vi "获取仪器仪表状态.vi"(11 "站号":u16(ring)=3 items=["总磷"=1, "总氮"=2, "氨氮"=3, "CODMn"=21, "CODcr"=22]) -> (3 "工作状态":T1(ring))   [LabVIEW 2016, in "质控单元V1.lvlib"]
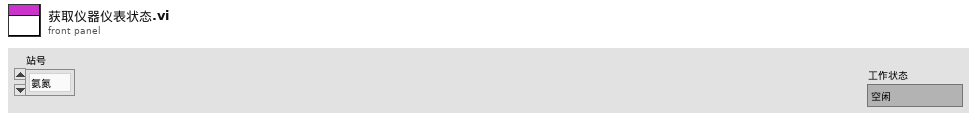
[diagram p1: front panel]
types:
  T1 = enum16{"空闲", "水样测试", "标样核查", "零点核查", "跨度核查", "空白测试", "平行样测试", "加标回收", "空白校准", "标样校准", "初始化（清洗）"}
  T2 = cluster{"系统时间":timestamp, "工作状态":enum16{"空闲", "水样测试", "标样核查", "零点核查", "跨度核查", "空白测试", "平行样测试", "加标回收", "空白校准", "标样校准", "初始化（清洗）"}, "测量模式":enum16{"待机", "连续模式", "周期模式", "定点模式", "受控模式", "手动模式"}, "告警代码":u16, "故障代码":u16, "日志代码":u16, "软件版本":u16}
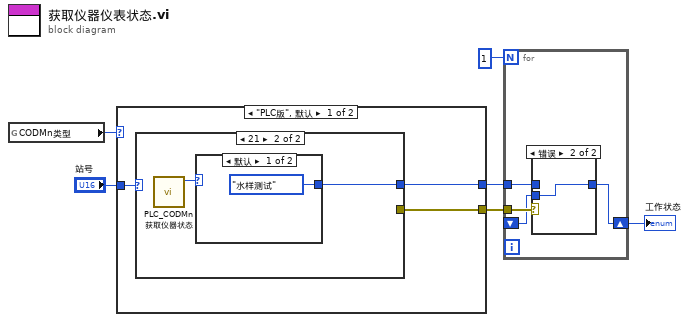
[diagram p0: block diagram]
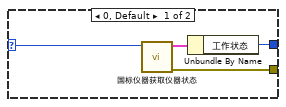
[diagram p3: hidden frame]
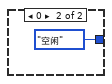
[diagram p4: hidden frame]
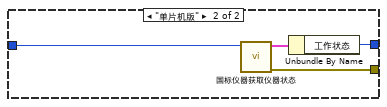
[diagram p5: hidden frame]
diagram:
  n1 = global read "系统交互.vi" "CODMn类型"() -> (w5:enum16{"PLC版", "单片机版"})
  n2 = case shown="\"PLC版\", 默认" w5 {
    tunnel: "站号" -> [w9 w21]
    tunnel: [w8 w20] -> w3
    tunnel: [w7 w18] -> w4
    frame "PLC版", Default {
      n3 = case shown="21" w9 {
        selector: w9 -> [w13 _]
        tunnel: [w11 w14] -> w8
        tunnel: [w10 _] -> w7
        frame 0, Default {
          n4 = call "国标仪器获取仪器状态.vi"("站号"=w13) -> ("error out"=w10:errorcluster, "状态告警区"=w12:T2)  [unwired: 9 in]
          n5 = Unbundle By Name(w12) -> ("工作状态"=w11:T1)
        }
        frame 21 {
          n6 = call "PLC_CODMn 获取仪器状态.vi"() -> ("PLC版_CODMn状态"=w15:u16)  [unwired: 11 in]
          n7 = case shown="默认" w15 {
            tunnel: [T1."水样测试" ("工作状态") T1."空闲" ("工作状态")] -> w14
            frame Default {
            }
            frame 0 {
            }
          }
        }
      }
    }
    frame "单片机版" {
      n8 = call "国标仪器获取仪器状态.vi"("站号"=w21) -> ("error out"=w18:errorcluster, "状态告警区"=w19:T2)  [unwired: 9 in]
      n9 = Unbundle By Name(w19) -> ("工作状态"=w20:T1)
    }
  }
  n10 = for {
    N: 1 -> [_]
    tunnel: w4 -> [w25]
    shift-right: [w23] -> w2
    shift-left: _ -> [w24]
    tunnel: w3 -> [w22]
    n11 = case shown="错误" w25 {
      tunnel: w24 -> [_ w27]
      tunnel: [w26 w27] -> w23
      tunnel: w22 -> [w26 _]
      frame No Error {
      }
      frame Error {
      }
    }
  }
  "工作状态" <- w2
